vi "FindSubpanels.PathArray.vi"(6 "Append (F)":bool, 8 "error in":errorcluster, 10 "Subpanel List":path[](array[path]), 11 "SMO.UI.MAUI in":refnum<class "SMO.UI.MAUI.lvclass">) -> (0 "error out":errorcluster, 3 "SMO.UI.MAUI out":refnum<class "SMO.UI.MAUI.lvclass">)   [LabVIEW 2020, in "SMO.UI.MAUI.lvclass"]
uses:
  SMO.UI.MAUI.lvclass
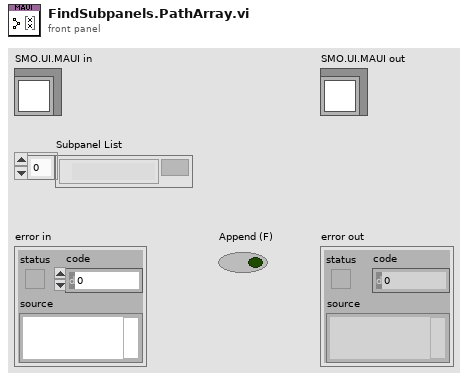
[diagram p1: front panel]
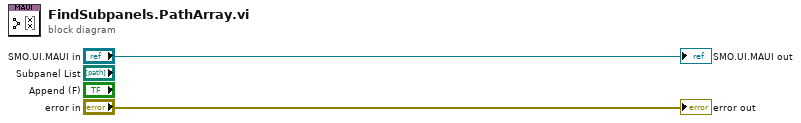
[diagram p0: block diagram]
diagram:
  "error out" <- "error in"
  "SMO.UI.MAUI out" <- "SMO.UI.MAUI in"
